vi "_008.vi"() -> ()   [LabVIEW 2024]
panel:
  in  "stop":bool
  in  "x":dbl
  out "Tank":dbl(slide) scale=0.0..20.0
  in  "Slide":dbl(slide) scale=0.0..10.0
  # "Structures :"
  # "(While Loop)"
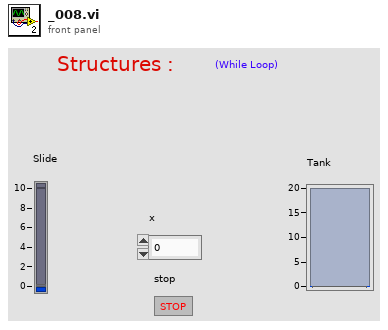
[diagram p1: front panel]
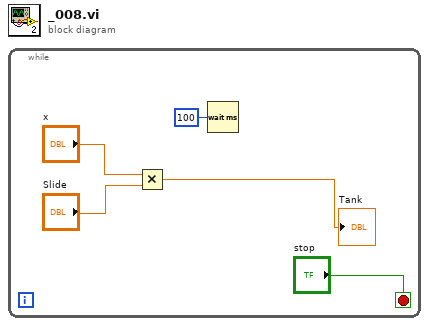
[diagram p0: block diagram]
diagram:
  n1 = while {
    stop <- "stop" stop-if-true
    n2 = Multiply(x="x", y="Slide") -> (x*y=→"Tank":dbl)
    n3 = Wait (ms)(milliseconds to wait=u32 100) -> ()  [unwired: 1 out]
  }
